vi "ConvertTo(UIMessage).vi"(8 "error in":errorcluster, 9 "Message Payload":variant) -> (0 "error out":errorcluster, 1 "UIMsg":T1)   [LabVIEW 2018]
doc: "Convert variant to DBL scalar\n\nBolder Software LLC"
uses:
  UIMessage.ctl
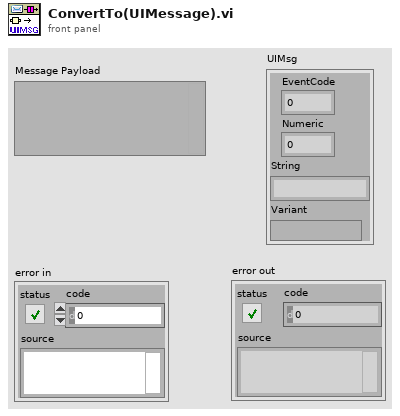
[diagram p1: front panel]
types:
  T1 = typedef "UIMessage.ctl" = cluster{"EventCode":i32, "Numeric":dbl, "String":string, "Variant":variant}
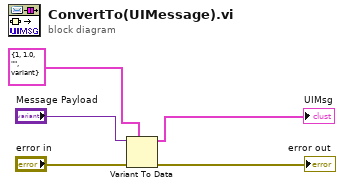
[diagram p0: block diagram]
diagram:
  n1 = Variant To Data(error in="error in", type=T1 {"EventCode"=1, "Numeric"=1.0, "String"="", "Variant"=variant} ("EZ-Zone Temp, Mode"), Variant="Message Payload") -> (data=→"UIMsg":T1, error out=→"error out":errorcluster)
